vi "Get Combination Index.vi"(10 "n":i32, 11 "m":i32) -> (2 "C(n,m)":i32, 3 "C(n,m) Items":i32[](array[numeric]))   [LabVIEW 2021, in "EDT Array.lvlib"]
uses:
  EDT Array.lvlib
  bbade539-64c7-496e-b2bf-67bf532cc53f.vi
  0207623e-f71f-464f-8a76-c2ad70ae0ada.vi
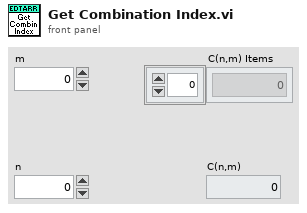
[diagram p1: front panel]
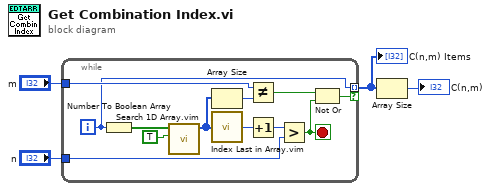
[diagram p0: block diagram]
diagram:
  n1 = while {
    tunnel: "m" -> [w15]
    tunnel: "n" -> [w14]
    tunnel: [w5] -> w2 mode=indexing if=w6
    i -> [w5]
    stop <- w7 stop-if-true
    n2 = Number To Boolean Array(number=w5) -> (Boolean array=w12:bool[])
    n3 = call "Search 1D Array.vim"("Element Data"=TRUE, "Array"=w12) -> ("Indices of Elements"=w10:i32[])  [unwired: 7 in]
    n4 = Array Size(array=w10) -> (size(s)=w11:i32)
    n5 = call "Index Last in Array.vim"("Array"=w10) -> ("Last Item"=w9:i32)
    n6 = Not Equal?(x=w15, y=w11) -> (x != y?=w16:bool)
    n7 = Increment(x=w9) -> (x+1=w8:i32)
    n8 = Greater?(x=w8, y=w14) -> (0:w7:bool)
    n9 = Not Or(1:w7, 2:w16) -> (0:w6:bool)
  }
  "C(n,m) Items" <- w2
  n10 = Array Size(array=w2) -> (size(s)=→"C(n,m)":i32)
